vi "API_Get Operational Configuration.vi"(8 "error in (no error)":errorcluster) -> (0 "error out":errorcluster, 1 "timed out?":bool, 3 "Tool OpCfg":T1={"Use Tool Cfg"=FALSE, "Use Tool Cal"=FALSE, "Fake Data?"=FALSE, "Mode"=-2, "Array Subset Length"=30, "nArrays to Read"=2, "Full Array Read Length"=500, "nSubarrays/Sensor"=0})   [LabVIEW 2015, in "Tool Module.lvlib"]
doc: "Returns the current state of the Tool Module Op Config cluster."
uses:
  Tool Module.lvlib
  Tool Config/_Tool Operation Config Cluster--typedef.ctl
  Tool Config/Tool Cfg.lvlib
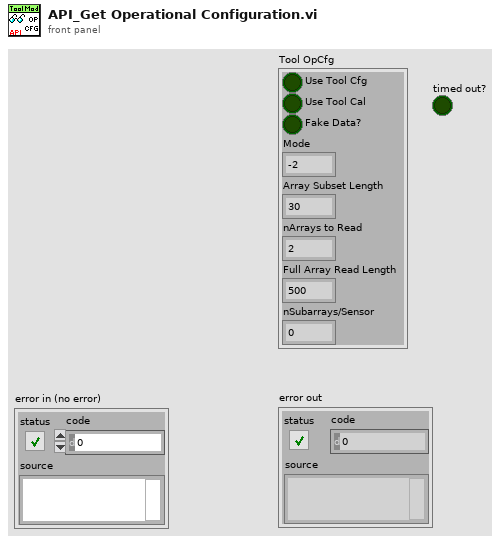
[diagram p1: front panel]
types:
  T1 = typedef "Tool Cfg.lvlib/_Tool Operation Config Cluster--typedef.ctl" = cluster{"Use Tool Cfg":bool, "Use Tool Cal":bool, "Fake Data?":bool, "Mode":i16, "Array Subset Length":i16, "nArrays to Read":i16, "Full Array Read Length":i16, "nSubarrays/Sensor":i16}
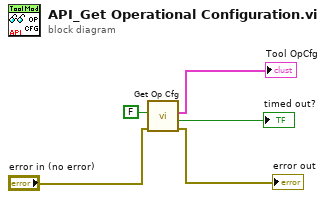
[diagram p0: block diagram]
diagram:
  n1 = call "Get Op Cfg.vi"("error in (no error)"="error in (no error)", "dummy"=FALSE) -> ("error out"=→"error out":errorcluster, "timed out?"=→"timed out?":bool, "Tool OpCfg"=→"Tool OpCfg":T1)  [unwired: 7 in]
